vi "802_11_b_g_n_16_to_JSON.vi"() -> ()   [LabVIEW 2019]
panel:
  out "JSON string":string
  in  "QAM Data":cluster{dbl[], dbl[]}
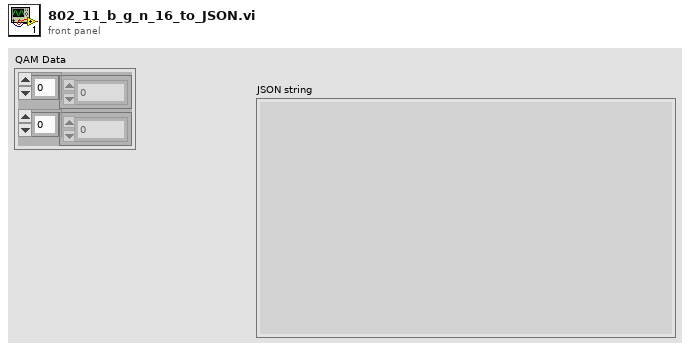
[diagram p1: front panel]
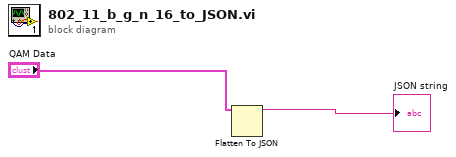
[diagram p0: block diagram]
diagram:
  n1 = Flatten To JSON(anything="QAM Data") -> (JSON string=→"JSON string":string)  [unwired: 2 in, 1 out]
